vi "tlc_Cue Module.vi"(5 "Number of Channels":cluster{"Rows":i32, "Columns":i32}, 6 "Command":T3, 7 "error in (no error)":errorcluster, 8 "Cue Input":T1={"Cue Name"="", "Wait Time (s)"=0, "Fade Time (s)"=1, "Follow Time (s)"=0, "Channels"=[]} {"Channels"."Intensität" min=0.0 max=100.0 step=1.0 format="%#.0f"}, 10 "Cue Index":i32 min=0) -> (0 "error out":errorcluster, 1 "Cue Output":T1 {"Channels"."Intensität" min=0.0 max=100.0 step=1.0 format="%#.0f"}, 2 "Number of Cues":i32)   [LabVIEW 2010]
doc: "Controls access to the Cue data."
uses:
  tlc_Cue_Information Command.ctl
  Controls/tlc_Cue_Information.ctl
  Controls/channel.ctl
panel:
  # "Output"
  # "Input"
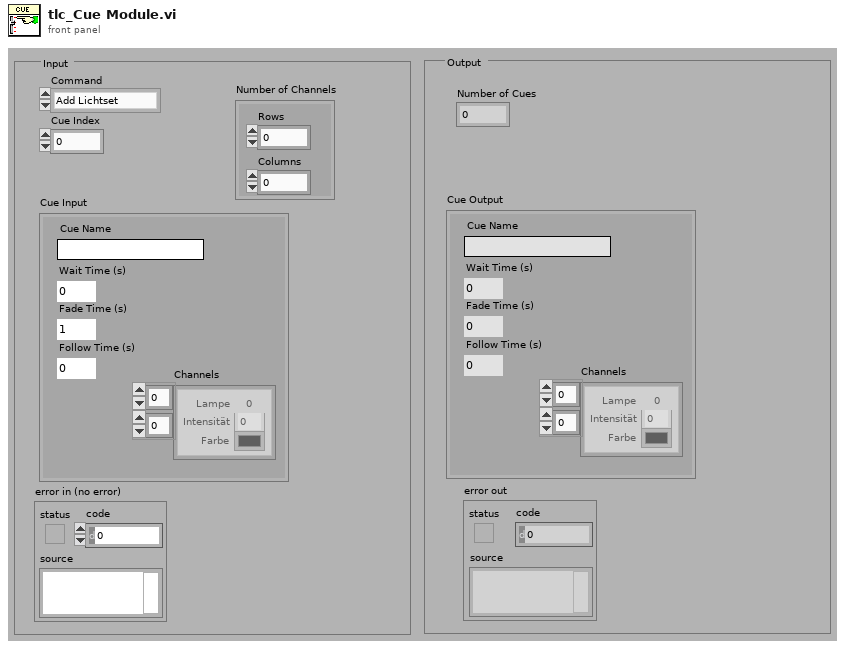
[diagram p1: front panel]
types:
  T1 = typedef "tlc_Cue_Information.ctl" = cluster{"Cue Name":string, "Wait Time (s)":u32, "Fade Time (s)":u32, "Follow Time (s)":u32, "Channels":T2[][]}
  T2 = typedef "channel.ctl" = cluster{"Intensität":dbl, " Farbe":u32, "Channel":i32}
  T3 = typedef "tlc_Cue_Information Command.ctl" = enum16{"Add Lichtset", "Get Lichtset Werte", "Set Lichtset Werte", "Get Anzahl Lichtersets", "Init", "Get Leeres Lichterset"}
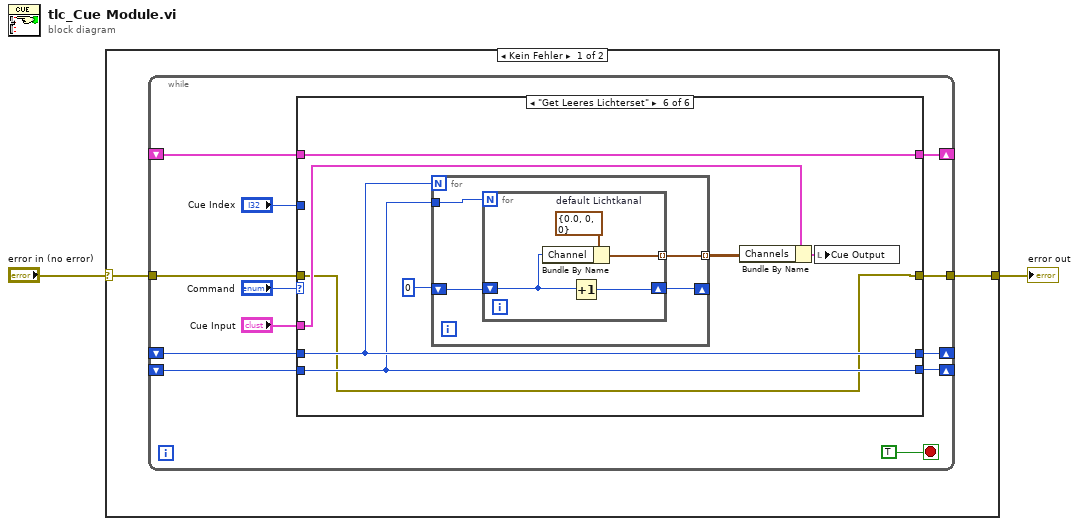
[diagram p0: block diagram]
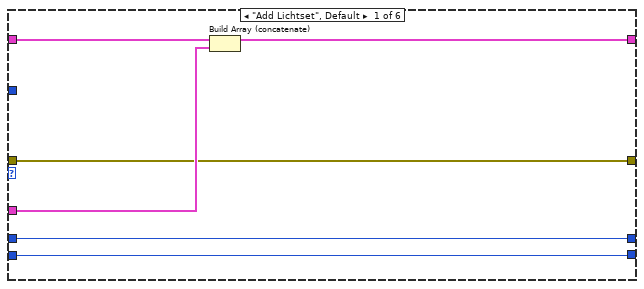
[diagram p2: hidden frame]
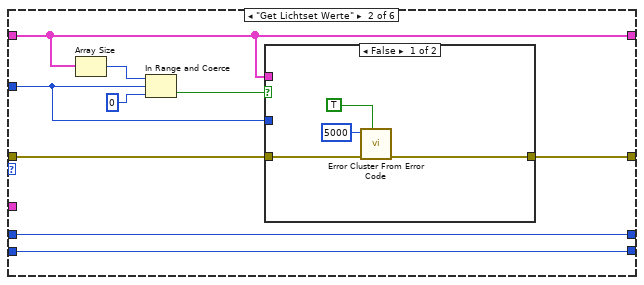
[diagram p3: hidden frame]
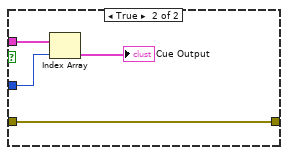
[diagram p4: hidden frame]
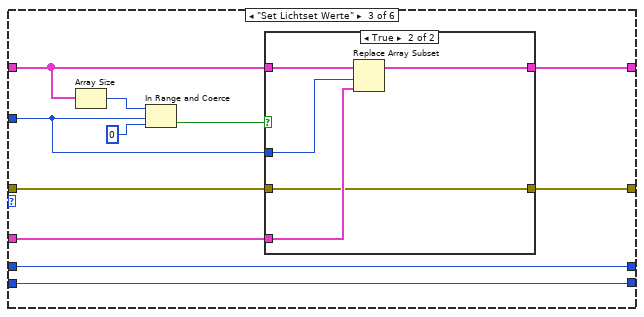
[diagram p5: hidden frame]
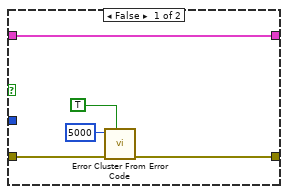
[diagram p6: hidden frame]
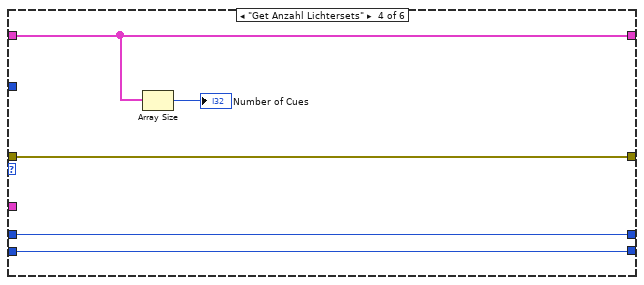
[diagram p7: hidden frame]
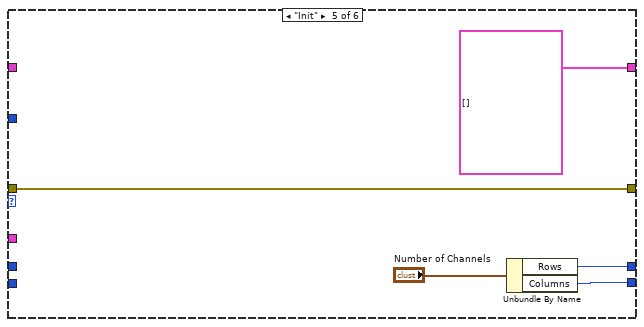
[diagram p8: hidden frame]
diagram:
  n1 = case shown="Kein Fehler" "error in (no error)" {
    selector: "error in (no error)" -> [w4 w87]
    tunnel: [w3 w87] -> w1
    frame No Error {
      n2 = while {
        shift-right: [w13] -> _
        shift-left: _ -> [w12]
        shift-right: [w10] -> _
        shift-left: _ -> [w8]
        shift-right: [w9] -> _
        shift-left: _ -> [w7]
        tunnel: w4 -> [w6]
        tunnel: [w5] -> w3
        stop <- TRUE stop-if-true
        n3 = case shown="\"Get Leeres Lichterset\"" "Command" {
          tunnel: "Cue Input" -> [w22 _ w49 _ _ w72]
          tunnel: [w21 w24 w50 w65 T1[] [] w75] -> w13
          tunnel: w12 -> [w20 w24 w45 w65 _ w75]
          tunnel: "Cue Index" -> [_ w23 w41 _ _ _]
          tunnel: [w19 w31 w48 w63 w68 w78] -> w10
          tunnel: [w18 w30 w47 w62 w67 w77] -> w9
          tunnel: w8 -> [w19 w31 w48 w63 _ w78]
          tunnel: w7 -> [w18 w30 w47 w62 _ w77]
          tunnel: [w17 w26 w44 w61 w66 w71] -> w5
          tunnel: w6 -> [w17 w27 w43 w61 w66 w71]
          frame "Add Lichtset", Default {
            n4 = Build Array (concatenate) "Build Array"(w20, w22) -> (w21:T1[])
          }
          frame "Get Lichtset Werte" {
            n5 = Array Size(array=w24) -> (size(s)=w25:i32)
            n6 = In Range and Coerce(upper limit=w25, x=w23, lower limit=0) -> (In Range?=w28:bool)  [unwired: 1 out]
            n7 = case shown="False" w28 {
              tunnel: w24 -> [_ w38]
              tunnel: w27 -> [w35 w37]
              tunnel: [w34 w37] -> w26
              tunnel: w23 -> [_ w36]
              frame False {
                n8 = call <vilib>:"Error Cluster From Error Code.vi"("show call chain? (False)"=TRUE, "error in (no error)"=w35, "error code (0)"=5000) -> ("error out"=w34:errorcluster)  [unwired: 6 in]
              }
              frame True {
                n9 = Index Array "Index Array"(array=w38, index=w36) -> (element=→"Cue Output":T1)
              }
            }
          }
          frame "Set Lichtset Werte" {
            n10 = Array Size(array=w45) -> (size(s)=w40:i32)
            n11 = In Range and Coerce(upper limit=w40, x=w41, lower limit=0) -> (In Range?=w42:bool)  [unwired: 1 out]
            n12 = case shown="True" w42 {
              tunnel: [w51 w60] -> w50
              tunnel: w49 -> [_ w59]
              tunnel: w45 -> [w51 w58]
              tunnel: [w52 w57] -> w44
              tunnel: w43 -> [w53 w57]
              tunnel: w41 -> [_ w56]
              frame False {
                n13 = call <vilib>:"Error Cluster From Error Code.vi"("show call chain? (False)"=TRUE, "error in (no error)"=w53, "error code (0)"=5000) -> ("error out"=w52:errorcluster)  [unwired: 6 in]
              }
              frame True {
                n14 = Replace Array Subset "Replace Array Subset"(array=w58, new element=w59, index=w56) -> (w60:T1[])
              }
            }
          }
          frame "Get Anzahl Lichtersets" {
            n15 = Array Size(array=w65) -> (size(s)=→"Number of Cues":i32)
          }
          frame "Init" {
            n16 = Unbundle By Name("Number of Channels") -> ("Rows"=w68:i32, "Columns"=w67:i32)
          }
          frame "Get Leeres Lichterset" {
            n17 = for {
              N: w78 -> [_]
              tunnel: w77 -> [w82]
              shift-right: [w79] -> _
              shift-left: 0 -> [w81]
              tunnel: [w80] -> w74 mode=indexing
              n18 = for {
                N: w82 -> [_]
                shift-right: [w85] -> w79
                shift-left: w81 -> [w84]
                tunnel: [w83] -> w80 mode=indexing
                w86 = T2 {"Intensität"=0.0, " Farbe"=0, "Channel"=0}  # default Lichtkanal
                n19 = Bundle By Name "Bundle By Name"(cluster=w86, "Channel"=w84) -> (w83:T2)
                n20 = Increment(x=w84) -> (x+1=w85:i32)
              }
            }
            n21 = Bundle By Name "Bundle By Name"(cluster=w72, "Channels"=w74) -> (w73:T1)
            n22 = local write "Cue Output"(w73) -> ()
          }
        }
      }
    }
    frame Error {
    }
  }
  "error out" <- w1
